vi "K2450Multilingual.vi"(7 "error in":errorcluster, 10 "VISA resource name":refnum<visa-resource-name>) -> (0 "Language":string, 1 "AutozeroOnce":string, 2 "Set Compliance":string, 3 "Set Source Level":string, 4 "Clear defbuffer1":string, 5 "error out":errorcluster {"code" format="%.0x"}, 6 "dup VISA Session":refnum<visa-resource-name>)   [LabVIEW 2025]
doc: "The VI sends *LANG? command to the specified VISA name. The VI does not test the model of the device with the VISA name. \nVI outputs are the language selected in the Keithley 2450 device TSP/SCPI/SCPI2400 and several often used (sets of) commands at the selected lenguage. The latter allows to avoid IF loops in critical parts of codes.\n\nAuthor: Scott Hannahs <sth@magnet.fsu.edu>\n\nThis software is licensed for use under the “MIT License\"\nCopyright (c) 2025 Scott Hannahs, sth@sth@magnet.sthnet.net\n\nPermission is hereby granted, free of charge, to any person obtaining a copy of this software and associated documentation files (the \"Software\"), to deal in the Software without restriction, including without limitation the rights to use, copy, modify, merge, publish, distribute, sublicense, and/or sell copies of the Software, and to permit persons to whom the Software is furnished to do so, subject to the following conditions: The above copyright notice and this permission notice shall be included in all copies or substantial portions of the Software.\n\nTHE SOFTWARE IS PROVIDED \"AS IS\", WITHOUT WARRANTY OF ANY KIND, EXPRESS OR IMPLIED, INCLUDING BUT NOT LIMITED TO THE WARRANTIES OF MERCHANTABILITY, FITNESS FOR A PARTICULAR PURPOSE AND NONINFRINGEMENT. IN NO EVENT SHALL THE AUTHORS OR COPYRIGHT HOLDERS BE LIABLE FOR ANY CLAIM, DAMAGES OR OTHER LIABILITY, WHETHER IN AN ACTION OF CONTRACT, TORT OR OTHERWISE, ARISING FROM, OUT OF OR IN CONNECTION WITH THE SOFTWARE OR THE USE OR OTHER DEALINGS IN THE SOFTWARE."
uses:
  <vilib>/Utility/error.llb/Trim Whitespace One-Sided.vi
panel:
  # "Commands:"
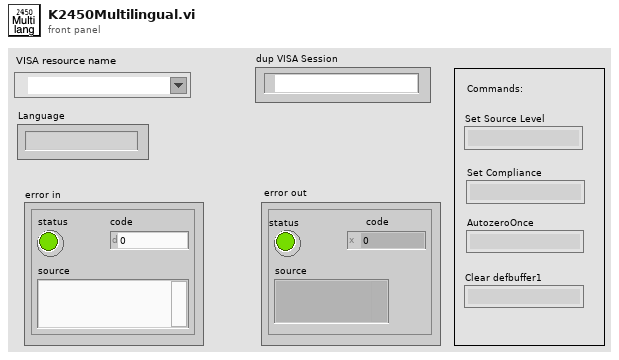
[diagram p1: front panel]
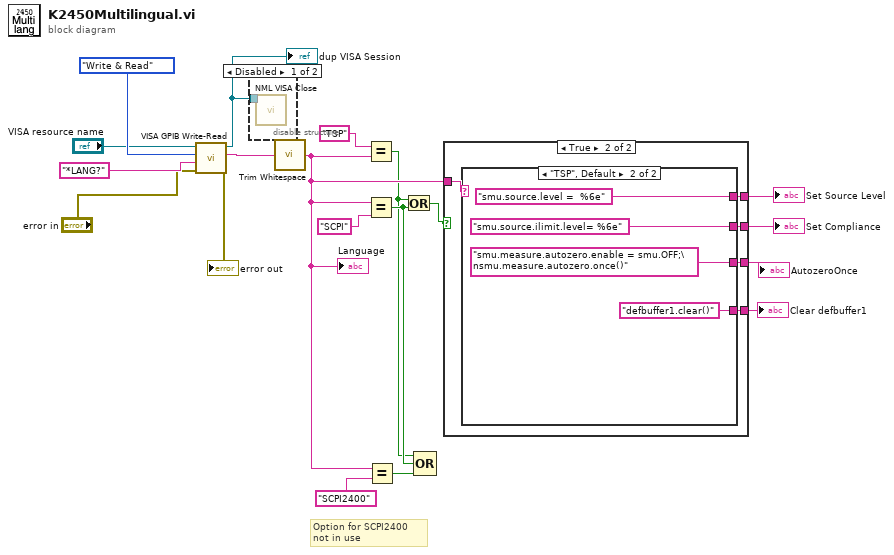
[diagram p0: block diagram]
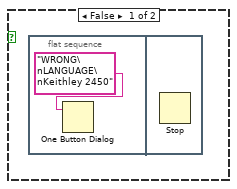
[diagram p3: hidden frame]
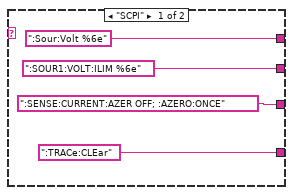
[diagram p4: hidden frame]
diagram:
  # "Option for SCPI2400 \nnot in use"
  n1 = call "VISA GPIB Write-Read.vi"("error in (no error)"="error in", "Command"="*LANG?", "Action"=enum16{"Write", "Read", "Write & Read"}."Write & Read", "VISA resource name"="VISA resource name") -> ("error out"=→"error out":errorcluster, "String Returned"=w14:string, "dup VISA Session"=w2:refnum<visa-resource-name>)  [unwired: 4 in, 1 out]
  "dup VISA Session" <- w2
  n2 = disable-structure shown="Disabled" {
    disable-tunnel: w2 -> [w20 _]
    frame Disabled {
      n3 = call "NML VISA Close.vi"("VISA resource name"=w20) -> ()  [unwired: 10 in, 1 out]
    }
    frame Enabled {
    }
  }
  n4 = call <vilib>:"Trim Whitespace.vi"("string"=w14) -> ("trimmed string"=w9:string)  [unwired: 1 in]
  "Language" <- w9
  n5 = Equal?(x="TSP" ("y"), y=w9) -> (x = y?=w6:bool)
  n6 = Equal?(x=w9, y="SCPI") -> (x = y?=w7:bool)
  n7 = Equal?(x=w9, y="SCPI2400") -> (x = y?=w8:bool)
  n8 = Or(x=w6, y=w7) -> (x .or. y?=w3:bool)
  n9 = Compound Arithmetic op=OR(w6, w7, w8) -> ()  [unwired: 1 out]
  n10 = case shown="True" w3 {
    tunnel: w9 -> [_ w26]
    tunnel: [_ w25] -> w12
    tunnel: [_ w24] -> w11
    tunnel: [_ w23] -> w5
    tunnel: [_ w22] -> w1
    frame False {
      n11 = flat-sequence {
        frame #0 {
          n12 = One Button Dialog(message="WRONG\nLANGUAGE\nKeithley 2450") -> ()  [unwired: 1 in, 1 out]
        }
        frame #1 {
          n13 = Stop() -> ()  [unwired: 1 in]
        }
      }
    }
    frame True {
      n14 = case shown="\"TSP\", Default" w26 {
        tunnel: [":Sour:Volt %6e" "smu.source.level =  %6e"] -> w25
        tunnel: [":SOUR1:VOLT:ILIM %6e" "smu.source.ilimit.level= %6e"] -> w24
        tunnel: [":SENSE:CURRENT:AZER OFF; :AZERO:ONCE" "smu.measure.autozero.enable = smu.OFF;\nsmu.measure.autozero.once()"] -> w23
        tunnel: [":TRACe:CLEar" "defbuffer1.clear()"] -> w22
        frame "SCPI" {
        }
        frame "TSP", Default {
        }
      }
    }
  }
  "Set Source Level" <- w12
  "Set Compliance" <- w11
  "AutozeroOnce" <- w5
  "Clear defbuffer1" <- w1
